vi "Read Messages.vi"(8 "error in":errorcluster, 11 "Communicator Worker in":refnum<class "Communicator Worker.lvclass">) -> (0 "error out":errorcluster, 3 "Communicator Worker out":refnum<class "Communicator Worker.lvclass">)   [LabVIEW 2025, in "Communicator Worker.lvlib" / "Communicator Worker.lvclass"]
uses:
  Communicator Worker.lvclass
  Communicator Worker.lvclass/Communicator Worker.ctl
  Interfaces/ICommunicate/ICommunicate.lvclass
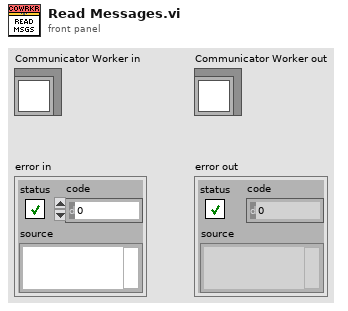
[diagram p1: front panel]
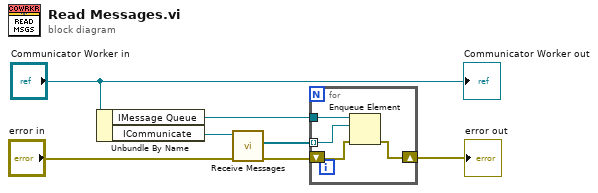
[diagram p0: block diagram]
diagram:
  n1 = Unbundle By Name("Communicator Worker in") -> ("IMessage Queue"=w3:refnum<queue>, "ICommunicate"=w6:refnum<class "ICommunicate.lvclass">)
  n2 = call-dynamic "Receive Messages.vi"("error in"="error in", "ICommunicate in"=w6) -> ("error out"=w2:errorcluster, "Messages"=w4:refnum<class "IMessage.lvclass">[])  [unwired: 7 in, 1 out]
  n3 = for {
    tunnel: w4 -> [w10] mode=indexing
    tunnel: w3 -> [w11]
    shift-right: [w8] -> w1
    shift-left: w2 -> [w9]
    n4 = Enqueue Element(queue=w11, element=w10, error in (no error)=w9) -> (error out=w8:errorcluster)  [unwired: 1 in, 2 out]
  }
  "error out" <- w1
  "Communicator Worker out" <- "Communicator Worker in"
